vi "Parse string to hex number.vi"(8 "error in (no error)":errorcluster, 11 "String":string) -> (0 "error out":errorcluster, 3 "Numeric":u32)   [LabVIEW 2019]
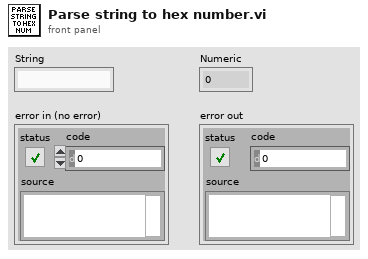
[diagram p1: front panel]
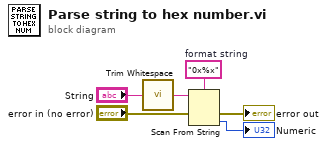
[diagram p0: block diagram]
diagram:
  w1 = "0x%x"  # format string
  n1 = call <vilib>:"Trim Whitespace.vi"("string"="String") -> ("trimmed string"=w4:string)  [unwired: 1 in]
  n2 = Scan From String(format string=w1, input string=w4, error in="error in (no error)") -> (error out=→"error out":errorcluster, output 1=→"Numeric":u32)  [unwired: 2 in, 2 out]
